vi "field sweep(SubVI).vi"(0 "data":refnum<queue>, 2 "Instrument Ref In":refnum<k24>, 4 "config":refnum<queue>, 5 "steps number":i32, 7 "ch str":string, 9 "Field":dbl=300.0, 11 "Mode":i32(ring) items=["Persistent", "Driven"], 12 "Resource In":refnum<visa-resource-name>, 13 "Field 2":dbl=300.0, 14 "Rate":dbl=10.0) -> (8 "错误输出":errorcluster)   [LabVIEW 2019, in "old.lvlib"]
uses:
  old.lvlib
  SubVI.lvlib
  lib/QDInstrument.dll
  config.ctl
  <vilib>/NI/Modbus Library/API/Master/Modbus Master.lvclass
  Instrument.ctl
panel:
  out "Field\nStatus 2":i32(ring) items=["MagnetUnknown"=0, "StablePersistent"=1, "WarmingSwitch"=2, "CoolingSwitch"=3, "StableDriven"=4, "Iterating"=5, "Charging"=6, "Discharging"=7, "CurrentError"=8, "MagnetFailure"=15]
  out "Field\nStatus":i32(ring) items=["MagnetUnknown"=0, "StablePersistent"=1, "WarmingSwitch"=2, "CoolingSwitch"=3, "StableDriven"=4, "Iterating"=5, "Charging"=6, "Discharging"=7, "CurrentError"=8, "MagnetFailure"=15]
  # "(真是通道1，假是通道2)"
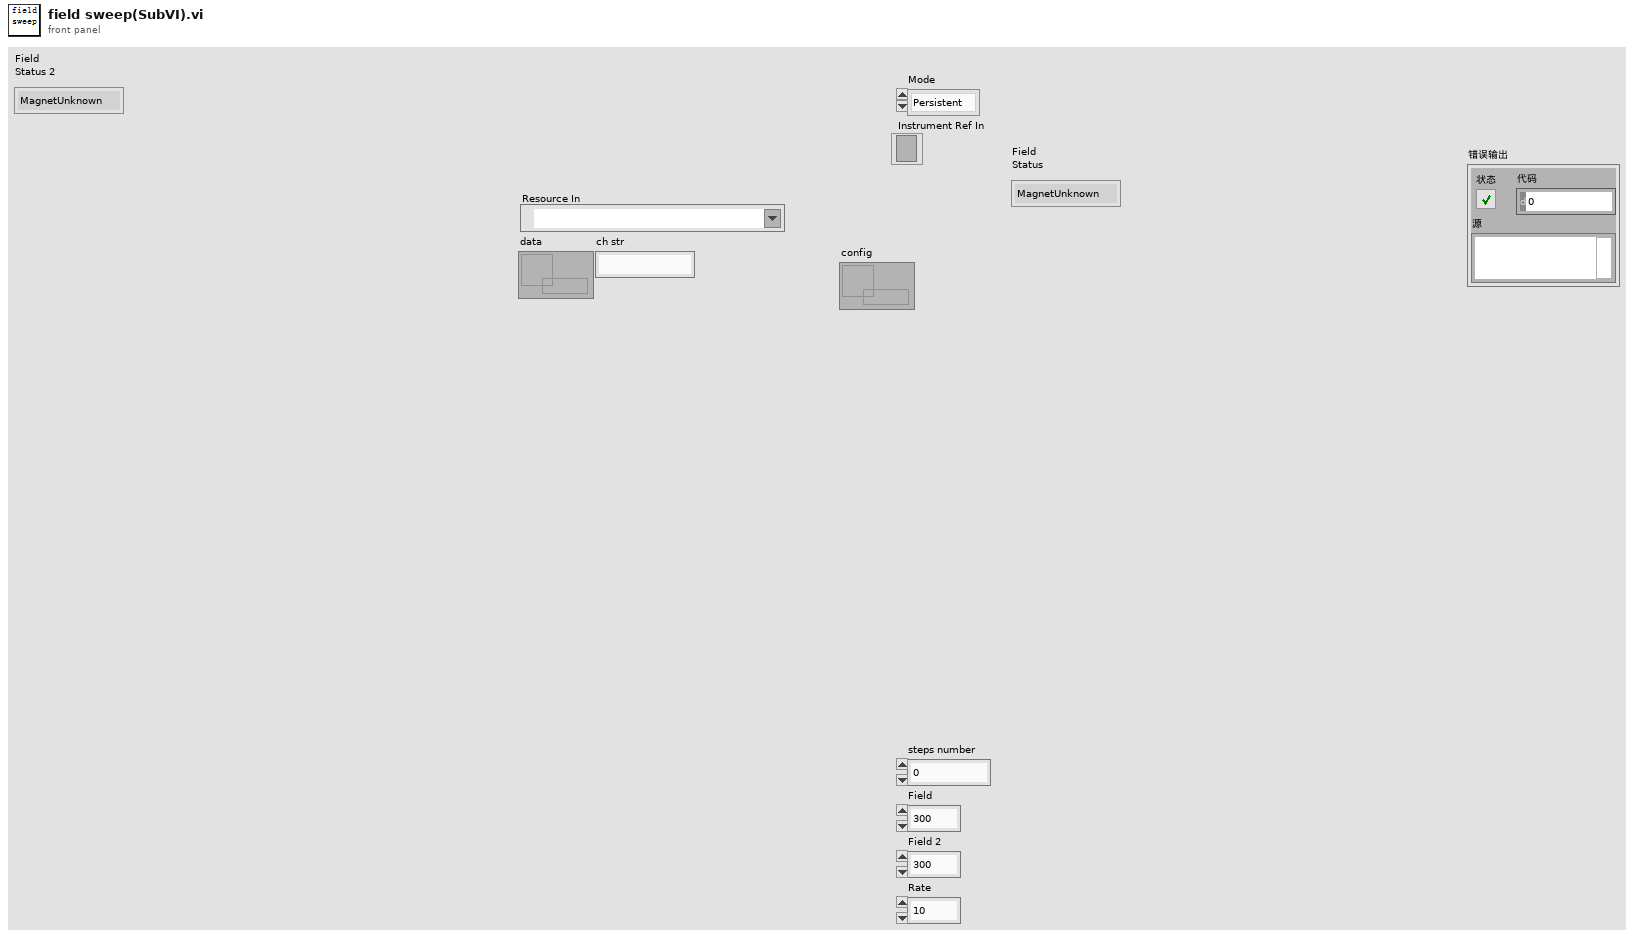
[diagram p1: front panel]
types:
  T1 = typedef "config.ctl" = cluster{"initialize":string, "6221":cluster{"6221 Resource":refnum<visa-resource-name>, "Delta status":bool}, "7001":cluster{"Ch":bool}, "SR830+6221":cluster{"source":u16, "阻抗":dbl, "量程入 4":i32, "量程入 3":i32, "量程入 2":i32, "量程入 1":i32, "电流":dbl, "SR830 2":bool, "SR830 3":bool, "SR830 4":bool, "SR830 1":bool, "VISA 1":refnum<visa-resource-name>, "VISA 2":refnum<visa-resource-name>, "VISA 3":refnum<visa-resource-name>, "VISA 4":refnum<visa-resource-name>, "量程":enum16{"量程每次测量会判定", "量程不变为设定值"}}, "2400":cluster{"2400":bool, "VISA":refnum<visa-resource-name>}, "ch":cluster{"ch str":string, "ch1":bool, "ch2":bool, "布尔":bool}, "error":bool, "数据文件路径":path, "log":cluster{"log路径":path, "log interval":dbl}, "Instrument":T2}
  T2 = typedef "Instrument.ctl" = cluster{"335 Resource":refnum<visa-resource-name>, "Input (0:A)":u16, "Instrument Type":i32, "quantum design":refnum<k24>, "Heater Output (1:1)":u16, "335state":refnum<vi>, "semaphore":T3, "TCP master instance":refnum<class "Modbus Master.lvclass">}
  T3 = typedef "Semaphore RefNum" = refnum<k1>
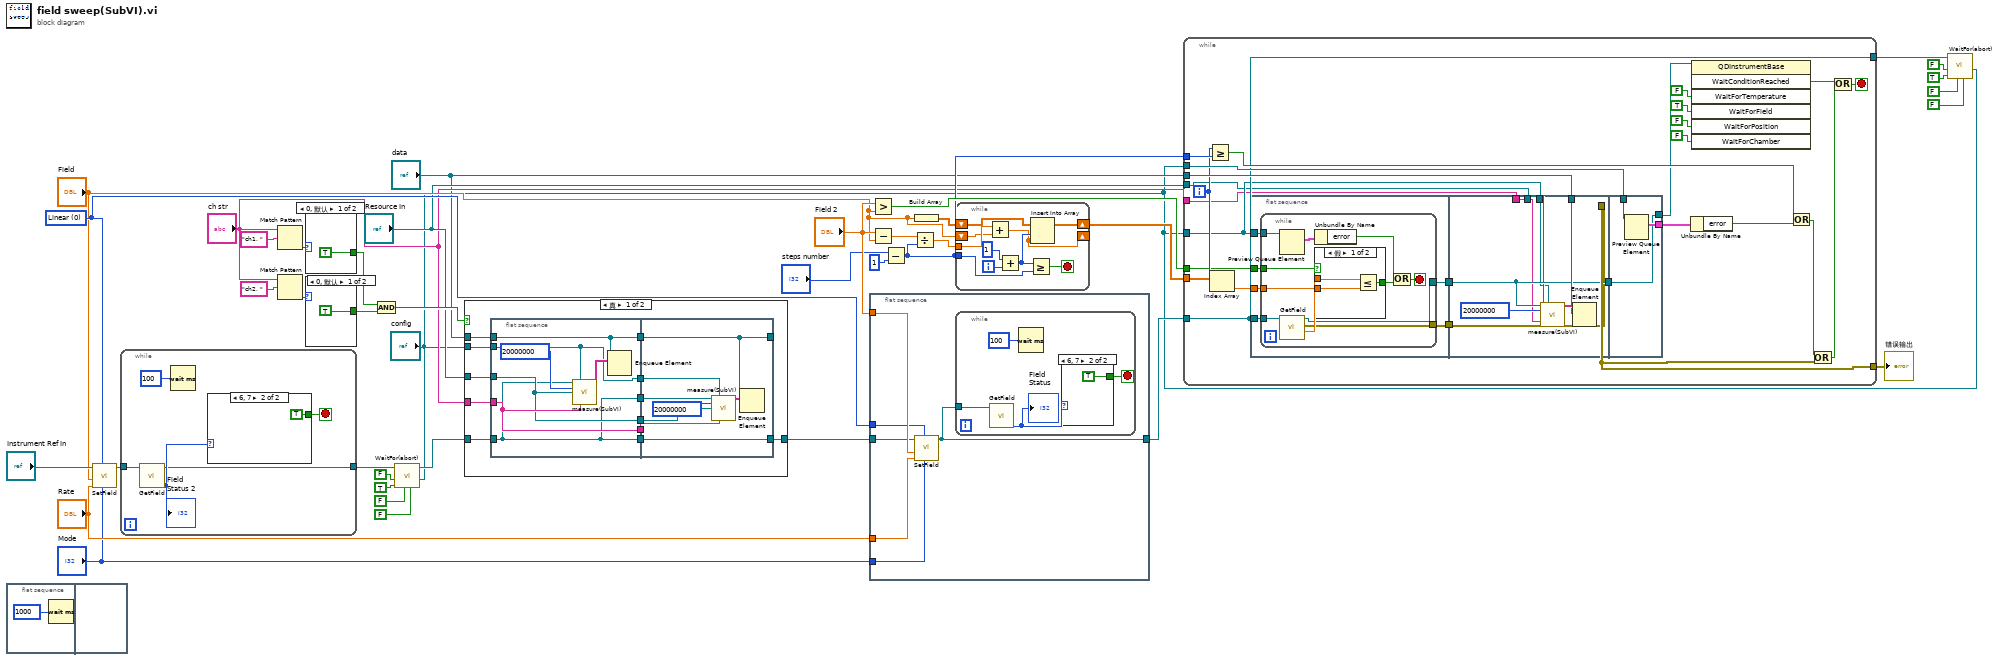
[diagram p0: block diagram]
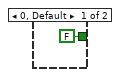
[diagram p2: hidden frame]
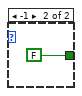
[diagram p3: hidden frame]
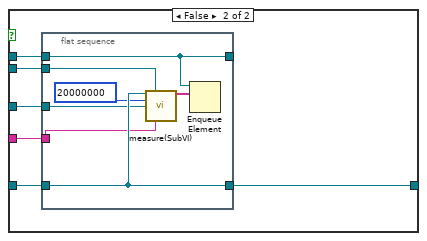
[diagram p4: hidden frame]
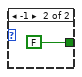
[diagram p5: hidden frame]
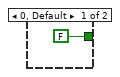
[diagram p6: hidden frame]
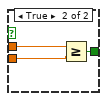
[diagram p7: hidden frame]
diagram:
  w35 = 0 items=["Linear", "NoOvershoot", "Oscillate"] ("Approach")
  n1 = flat-sequence {
    frame #0 {
      n2 = Wait (ms)(milliseconds to wait=u32 1000) -> ()  [unwired: 1 out]
    }
    frame #1 {
    }
  }
  n3 = call "SetField.vi"("Mode"="Mode", "Approach"=w35, "Rate"="Rate", "Field"="Field", "Instrument Ref In"="Instrument Ref In") -> ("Instrument Ref Out"=w2:refnum<k24>)  [unwired: 2 in, 2 out]
  n4 = while {
    tunnel: w2 -> [w46]
    tunnel: [w42] -> w1
    stop <- w44 stop-if-true
    n5 = call "GetField.vi"("Instrument Ref In"=w46) -> ("Field\nStatus"=w45:i32, "Instrument Ref Out"=w42:refnum<k24>)  [unwired: 4 in, 3 out]
    "Field\nStatus 2" <- w45
    n6 = Wait (ms)(milliseconds to wait=u32 100) -> ()  [unwired: 1 out]
    n7 = case shown="6, 7" w45 {
      tunnel: [FALSE TRUE] -> w44
      frame 0, Default {
      }
      frame 6, 7 {
      }
    }
  }
  n8 = Match Pattern(string="ch str", regular expression="ch1, " ("正则表达式")) -> (offset past match=w13:i32)  [unwired: 1 in, 3 out]
  n9 = Match Pattern(string="ch str", regular expression="ch2, " ("正则表达式")) -> (offset past match=w12:i32)  [unwired: 1 in, 3 out]
  n10 = case shown="0, 默认" w13 {
    tunnel: [TRUE FALSE] -> w11
    frame 0, Default {
    }
    frame -1 {
    }
  }
  n11 = case shown="0, 默认" w12 {
    tunnel: [TRUE FALSE] -> w10
    frame 0, Default {
    }
    frame -1 {
    }
  }
  n12 = And(x=w11, y=w10) -> (x .and. y?=w9:bool)
  n13 = call "WaitFor(abort).vi"("config"="config", "Wait For Chamber"=FALSE, "Wait For Position"=FALSE, "Wait For Field"=TRUE, "Wait For Temperature"=FALSE, "Instrument Ref In"=w1) -> ("Instrument Ref Out"=w8:refnum<k24>)  [unwired: 4 in, 1 out]
  n14 = case shown="真" w9 {
    tunnel: w8 -> [w64 w85]
    tunnel: "Resource In" -> [w63 w84]
    tunnel: "ch str" -> [w62 w83]
    tunnel: "data" -> [w61 w82]
    tunnel: "config" -> [w60 w81]
    tunnel: [w59 w80] -> w4
    frame True {
      n15 = flat-sequence {
        tunnel: w64 -> [w65]
        tunnel: w63 -> [w66]
        tunnel: w62 -> [w67]
        tunnel: w61 -> [w69]
        tunnel: w60 -> [w68]
        tunnel: [w65] -> w58
        tunnel: [w69] -> w57
        tunnel: [w68] -> w56
        tunnel: [w67] -> w55
        tunnel: [w66] -> w54
        tunnel: [w65] -> w53
        tunnel: [w72] -> _
        tunnel: [w79] -> w59
        tunnel: w58 -> [w79]
        tunnel: w57 -> [w72]
        tunnel: w56 -> [w76]
        tunnel: w55 -> [w75]
        tunnel: w54 -> [w74]
        tunnel: w53 -> [w73]
        frame #0 {
          n16 = call "measure(SubVI).vi"(0:w65, "config"=w68, 5:u32 20000000 ("Timeout (20000 ms)"), 7:w66, 12:w67) -> ("data"=w70:string[])  [unwired: 9 in, 1 out]
          n17 = Enqueue Element(queue=w69, element=w70) -> ()  [unwired: 2 in, 3 out]
        }
        frame #1 {
          n18 = call "measure(SubVI).vi"(0:w73, "config"=w76, 5:u32 20000000 ("Timeout (20000 ms)"), 7:w74, 12:w75) -> ("data"=w78:string[])  [unwired: 9 in, 1 out]
          n19 = Enqueue Element(queue=w72, element=w78) -> ()  [unwired: 2 in, 3 out]
        }
      }
    }
    frame False {
      n20 = flat-sequence {
        tunnel: w85 -> [w92]
        tunnel: [w92] -> w80
        tunnel: w84 -> [w90]
        tunnel: w83 -> [w89]
        tunnel: [w87] -> _
        tunnel: w82 -> [w87]
        tunnel: w81 -> [w86]
        frame #0 {
          n21 = call "measure(SubVI).vi"(0:w92, "config"=w86, 5:u32 20000000 ("Timeout (20000 ms)"), 7:w90, 12:w89) -> ("data"=w88:string[])  [unwired: 9 in, 1 out]
          n22 = Enqueue Element(queue=w87, element=w88) -> ()  [unwired: 2 in, 3 out]
        }
      }
    }
  }
  n23 = flat-sequence {
    tunnel: "Field 2" -> [w98]
    tunnel: "Rate" -> [w97]
    tunnel: w35 -> [w96]
    tunnel: "Mode" -> [w95]
    tunnel: [w93] -> w29
    tunnel: w4 -> [w94]
    frame #0 {
      n24 = call "SetField.vi"("Mode"=w95, "Approach"=w96, "Rate"=w97, "Field"=w98, "Instrument Ref In"=w94) -> ("Instrument Ref Out"=w93:refnum<k24>)  [unwired: 2 in, 2 out]
      n25 = while {
        tunnel: w93 -> [w102]
        stop <- w100 stop-if-true
        n26 = call "GetField.vi"("Instrument Ref In"=w102) -> ("Field\nStatus"=w101:i32)  [unwired: 4 in, 4 out]
        "Field\nStatus" <- w101
        n27 = Wait (ms)(milliseconds to wait=u32 100) -> ()  [unwired: 1 out]
        n28 = case shown="6, 7" w101 {
          tunnel: [FALSE TRUE] -> w100
          frame 0, Default {
          }
          frame 6, 7 {
          }
        }
      }
    }
  }
  n29 = Greater?(x="Field 2", y="Field") -> (0:w31:bool)
  n30 = Subtract(x="Field 2", y="Field") -> (x-y=w40:dbl)
  n31 = Subtract(x="steps number", y=1) -> (x-y=w20:i32)
  n32 = Divide(x=w40, y=w20) -> (x/y=w38:dbl)
  n33 = Build Array("Field") -> (w39:dbl[])
  n34 = while {
    shift-right: [w114] -> w33
    shift-left: w39 -> [w113]
    tunnel: w38 -> [w108]
    tunnel: w20 -> [w107]
    shift-right: [w106] -> _
    shift-left: "Field" -> [w105]
    i -> [w112]
    stop <- w109 stop-if-true
    n35 = Add(x=w108, y=w105) -> (x+y=w106:dbl)
    n36 = Add(x=1, y=w112) -> (x+y=w110:i32)
    n37 = Greater Or Equal?(x=w110, y=w107) -> (x >= y?=w109:bool)
    n38 = Insert Into Array(array=w113, index=w110, new element=w106) -> (w114:dbl[])
  }
  n39 = while {
    tunnel: w33 -> [w141]
    tunnel: w20 -> [w136]
    tunnel: "data" -> [w139]
    tunnel: "config" -> [w138]
    tunnel: w29 -> [w132]
    tunnel: w31 -> [w134]
    tunnel: [w132] -> w24
    tunnel: "config" -> [w131]
    tunnel: [w129] -> w23
    tunnel: "Resource In" -> [w118]
    tunnel: "ch str" -> [w117]
    i -> [w135]
    stop <- w119 stop-if-true
    n40 = Greater Or Equal?(x=w135, y=w136) -> (x >= y?=w137:bool)
    n41 = Index Array(array=w141, index=w135) -> (element=w133:dbl)
    n42 = flat-sequence {
      tunnel: [w144] -> w140
      tunnel: w132 -> [w147]
      tunnel: w134 -> [w146]
      tunnel: w133 -> [w145]
      tunnel: w131 -> [w143]
      tunnel: [w142] -> w130
      tunnel: w140 -> [w172]
      tunnel: w139 -> [w174]
      tunnel: w131 -> [w169]
      tunnel: w130 -> [w170]
      tunnel: [w167] -> w129
      tunnel: [w172] -> w122
      tunnel: w118 -> [w171]
      tunnel: w117 -> [w165]
      tunnel: w138 -> [w177]
      tunnel: [w176] -> w116
      tunnel: [w175] -> w123
      tunnel: w122 -> [w175]
      frame #0 {
        n43 = while {
          tunnel: w147 -> [w156]
          tunnel: w146 -> [w158]
          tunnel: w145 -> [w157]
          tunnel: [w150] -> w144
          tunnel: w143 -> [w154]
          tunnel: [w151] -> w142
          stop <- w152 stop-if-true
          n44 = Preview Queue Element(queue=w154) -> (element=w149:T1)  [unwired: 2 in, 3 out]
          n45 = call "GetField.vi"("Instrument Ref In"=w156) -> ("Field"=w155:dbl, "error out"=w151:errorcluster, "Instrument Ref Out"=w150:refnum<k24>)  [unwired: 4 in, 2 out]
          n46 = Unbundle By Name(w149) -> ("error"=w148:bool)
          n47 = case shown="假" w158 {
            tunnel: w155 -> [w161 w164]
            tunnel: w157 -> [w160 w163]
            tunnel: [w159 w162] -> w153
            frame False {
              n48 = Less Or Equal?(x=w161, y=w160) -> (x <= y?=w159:bool)
            }
            frame True {
              n49 = Greater Or Equal?(x=w164, y=w163) -> (x >= y?=w162:bool)
            }
          }
          n50 = Or(x=w148, y=w153) -> (x .or. y?=w152:bool)
        }
      }
      frame #1 {
        n51 = call "measure(SubVI).vi"(0:w172, "config"=w169, 5:u32 20000000 ("Timeout (20000 ms)"), 7:w171, "error in (no error)"=w170, 12:w165) -> ("data"=w173:string[], "error out"=w168:errorcluster)  [unwired: 8 in]
        n52 = Enqueue Element(queue=w174, element=w173, error in (no error)=w168) -> (error out=w167:errorcluster)  [unwired: 1 in, 2 out]
      }
      frame #2 {
        n53 = Preview Queue Element(queue=w177) -> (element=w176:T1)  [unwired: 2 in, 3 out]
      }
    }
    n54 = Unbundle By Name(w116) -> ("error"=w115:bool)
    n55 = invoke class="QDInstrumentBase" method="WaitConditionReached"(reference=w123, "WaitForTemperature"=FALSE, "WaitForField"=TRUE, "WaitForPosition"=FALSE, "WaitForChamber"=FALSE) -> ("WaitConditionReached"=w121:bool)  [unwired: 2 in, 6 out]
    n56 = Or(x=w137, y=w115) -> (x .or. y?=w128:bool)
    n57 = Or(x=w128, y=w129) -> (x .or. y?=w120:bool)
    n58 = Or(x=w121, y=w120) -> (x .or. y?=w119:bool)
  }
  "错误输出" <- w23
  n59 = call "WaitFor(abort).vi"("config"="config", "Wait For Chamber"=FALSE, "Wait For Position"=FALSE, "Wait For Field"=TRUE, "Wait For Temperature"=FALSE, "Instrument Ref In"=w24) -> ()  [unwired: 4 in, 2 out]
